vi "Get Config Value.vi"(8 "error in (no error)":errorcluster, 9 "Default":string, 10 "Name":string, 11 "Resource in":refnum<class "Resource.lvclass">) -> (0 "error out":errorcluster, 1 "Not Found?":bool, 2 "Value":string, 3 "Resource out":refnum<class "Resource.lvclass">)   [LabVIEW 2020, in "PicoG-Core.lvlib" / "Resource.lvclass"]
uses:
  Resource.lvclass
  Resource.lvclass/Resource.ctl
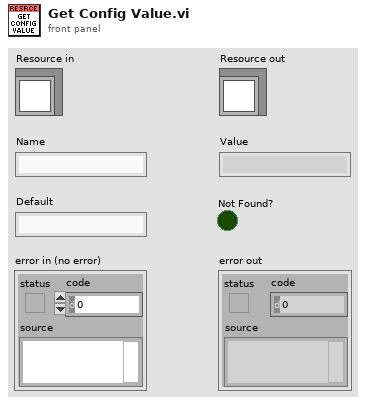
[diagram p1: front panel]
types:
  T1 = typedef "PicoG-Core.lvlib/Resource.lvclass/Ref Data.ctl" = cluster{"Config":map{string, string}, "Stream":refnum<class "Stream.lvclass">}
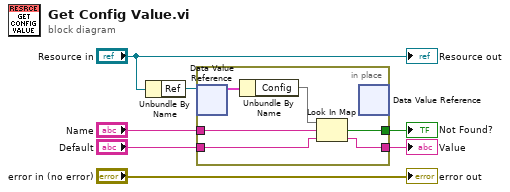
[diagram p0: block diagram]
diagram:
  n1 = Unbundle By Name("Resource in") -> ("Ref"=w1:refnum<data-value>)
  n2 = in-place {
    in-place-border: "Name" -> [w13]
    in-place-border: "Default" -> [w12]
    in-place-border: [w11] -> w3
    in-place-border: [w10] -> w2
    n3 = in-place-dvr #1(w1) -> (w9:T1)  [unwired: 1 out]
    n4 = Unbundle By Name(w9) -> ("Config"=w8:map{string, string})
    n5 = Look In Map(map=w8, key=w13, default value=w12) -> (key not found?=w11:bool, value=w10:string)
    n6 = in-place-dvr #1() -> ()  [unwired: 1 in, 2 out]
  }
  "Value" <- w2
  "Not Found?" <- w3
  "error out" <- "error in (no error)"
  "Resource out" <- "Resource in"
